vi "Close.vi"(8 "error in":errorcluster, 11 "VISA in":refnum<visa-resource-name>) -> (0 "error out":errorcluster)   [LabVIEW 2016, in "Serial_G.lvlib"]
doc: "Close VISA"
uses:
  Serial_G.lvlib
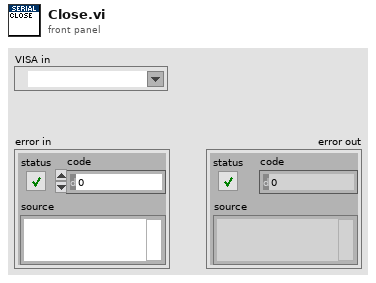
[diagram p1: front panel]
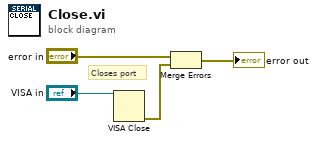
[diagram p0: block diagram]
diagram:
  # "Closes port"
  n1 = VISA Close(VISA resource name="VISA in") -> (error out=w1:errorcluster)  [unwired: 1 in]
  n2 = Merge Errors("error in", w1) -> (→"error out":errorcluster)
